vi "0 - 10 Solve Equations.vi"() -> ()   [LabVIEW 2012]
panel:
  out "Y1 Y2 Waveform Chart":cluster{"Y1":dbl, "Y2":dbl}(graph)
  in  "B Value":dbl
  in  "M Value":dbl
  out "Y2 Value":dbl
  out "Y1 Value":dbl
  in  "X Value":dbl min=0.0 max=10.0 step=1.0
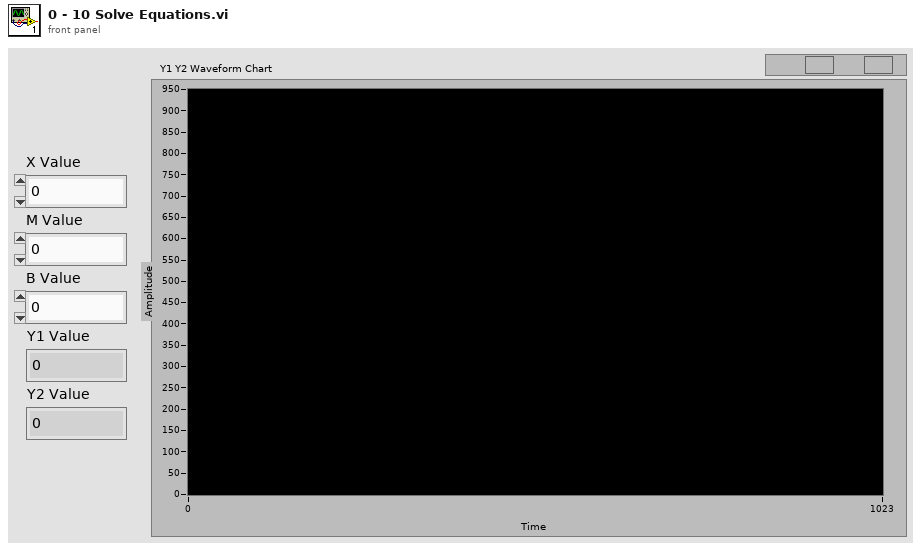
[diagram p1: front panel]
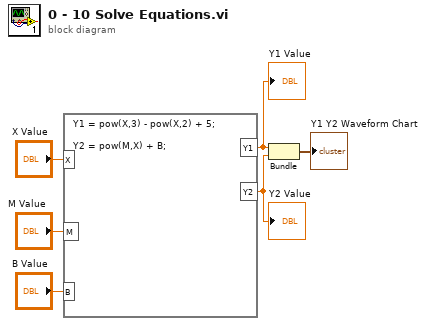
[diagram p0: block diagram]
diagram:
  n1 = formula code="Y1 = pow(X,3) - pow(X,2) + 5;\n\nY2 = pow(M,X) + B;"("X"="X Value", "M"="M Value", "B"="B Value") -> ("Y1"=w3:dbl, "Y2"=w2:dbl)
  "Y1 Value" <- w3
  "Y2 Value" <- w2
  n2 = Bundle("Y1"=w3, "Y2"=w2) -> (→"Y1 Y2 Waveform Chart":cluster{"Y1":dbl, "Y2":dbl})  [unwired: 1 in]
